vi "Do.vi"(8 "error in (no error)":errorcluster, 10 "Actor in":refnum<class "Actor.lvclass">, 11 "Launch Nested Actor Msg":refnum<class "Launch Nested Actor Msg.lvclass">) -> (0 "error out":errorcluster, 2 "Actor out":refnum<class "Actor.lvclass">)   [LabVIEW 2020, in "Actor Framework.lvlib" / "Launch Nested Actor Msg.lvclass"]
doc: "(<B>Filename</B>: Actor Framework.lvlib:Message.lvclass:Do.vi)\n\nDefines what a message does when it is received by an actor. Generally, a message instructs an actor to invoke one of its methods.\n\nBy default, this method does nothing. A child class must override it to define behavior. Create a child class by using the Actor Framework Message Maker dialog box."
uses:
  Launch Nested Actor Msg.lvclass
  Actor/Actor.lvclass
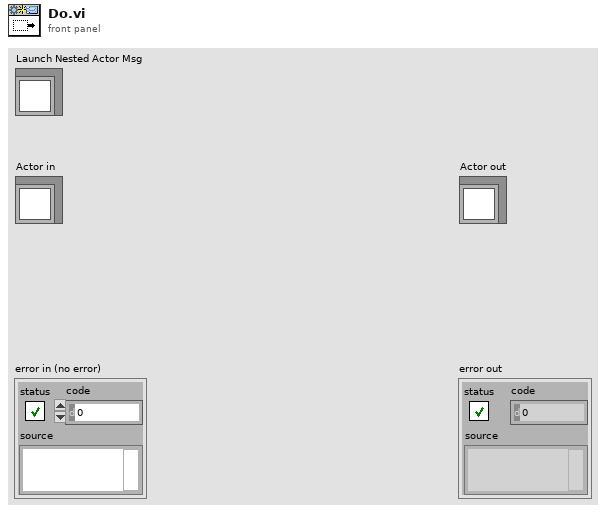
[diagram p1: front panel]
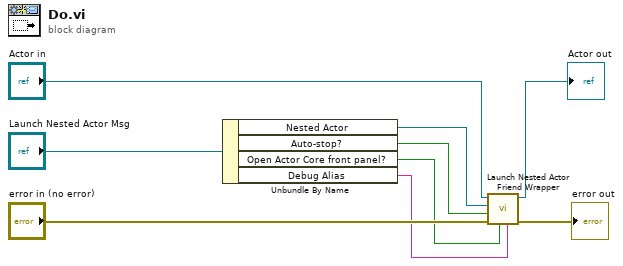
[diagram p0: block diagram]
diagram:
  n1 = Unbundle By Name("Launch Nested Actor Msg") -> ("Nested Actor"=w4:refnum<class "Actor.lvclass">, "Auto-stop?"=w3:bool, "Open Actor Core front panel?"=w2:bool, "Debug Alias"=w1:string)
  n2 = call "Launch Nested Actor Friend Wrapper.vi"("Debug Alias"=w1, "Open Actor Core front panel? (F)"=w2, "error in (no error)"="error in (no error)", "Auto-stop? (T)"=w3, "Nested Actor"=w4, "Caller Actor in"="Actor in") -> ("error out"=→"error out":errorcluster, "Caller Actor out"=→"Actor out":refnum<class "Actor.lvclass">)  [unwired: 3 in, 1 out]
